vi "Reconstruct Installation Directory.vi"(10 "Build Type":string, 11 "Aliased Installation Path":path) -> (2 "NIPKG Directory":path, 3 "Real Installation Path":path)   [LabVIEW 2019, in "NIPKG Packager.lvclass"]
uses:
  NIPKG Packager.lvclass
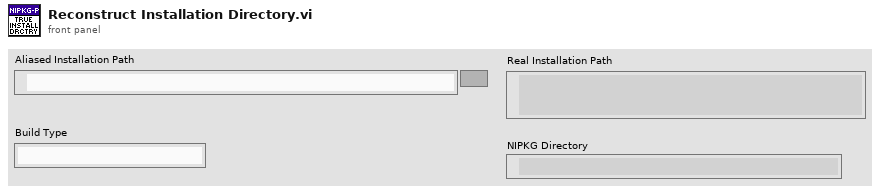
[diagram p1: front panel]
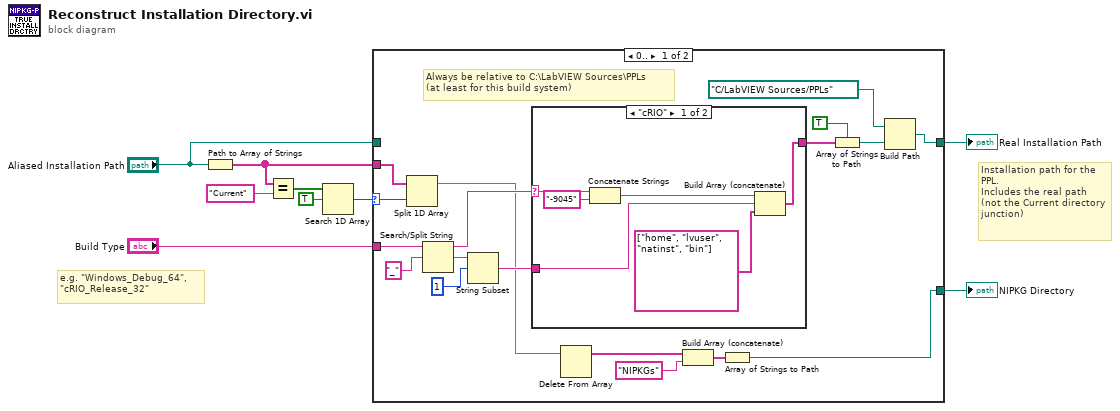
[diagram p0: block diagram]
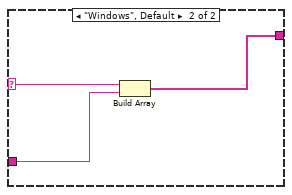
[diagram p2: hidden frame]
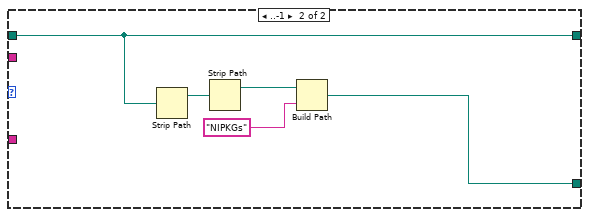
[diagram p3: hidden frame]
diagram:
  # "e.g. \"Windows_Debug_64\", \"cRIO_Release_32\""
  # "Installation path for the PPL.\nIncludes the real path (not the Current directory junction)"
  n1 = Path to Array of Strings(0:"Aliased Installation Path") -> (2:w3:string[])  [unwired: 1 out]
  n2 = Equal?(x=w3, y="Current") -> (x = y?=w8:bool[])
  n3 = Search 1D Array(1D array=w8, element=TRUE) -> (index of element=w6:i32)  [unwired: 1 in]
  n4 = case shown="0.." w6 {
    selector: w6 -> [w26 _]
    tunnel: [w11 w37] -> w5
    tunnel: "Build Type" -> [w24 _]
    tunnel: w3 -> [w27 _]
    tunnel: [w14 w38] -> w2
    tunnel: "Aliased Installation Path" -> [_ w37]
    frame 0.. {
      # "Always be relative to C:\\LabVIEW Sources\\PPLs\n(at least for this build system)"
      n5 = Split 1D Array(array=w27, index=w26) -> (first subarray=w18:string[])  [unwired: 1 out]
      n6 = Search/Split String(string=w24, search string/char (-)="_" ("delimiter")) -> (substring before match=w23:string, match + rest of string=w20:string)  [unwired: 1 in, 1 out]
      n7 = String Subset(string=w20, offset (0)=1) -> (substring=w19:string)  [unwired: 1 in]
      n8 = case shown="\"cRIO\"" w23 {
        selector: w23 -> [w32 w36]
        tunnel: [w28 w35] -> w22
        tunnel: w19 -> [w29 w34]
        frame "cRIO" {
          n9 = Concatenate Strings(w32, "-9045" ("string")) -> (w30:string)
          n10 = Build Array (concatenate)(w30, w29, string[] ["home", "lvuser", "natinst", "bin"] ("string")) -> (w28:string[])
        }
        frame "Windows", Default {
          n11 = Build Array(w36, w34) -> (w35:string[])
        }
      }
      n12 = Delete From Array(array=w18) -> (array with subset deleted=w17:string[])  [unwired: 2 in, 1 out]
      n13 = Build Array (concatenate)(w17, "NIPKGs") -> (w15:string[])
      n14 = Array of Strings to Path(0:w15) -> (2:w14:path)  [unwired: 1 in]
      n15 = Array of Strings to Path(0:w22, 1:TRUE ("relative")) -> (2:w12:path)
      n16 = Build Path(base path=path "C:/LabVIEW Sources/PPLs", name or relative path=w12) -> (appended path=w11:path)
    }
    frame ..-1 {
      n17 = Strip Path(path=w37) -> (stripped path=w41:path)  [unwired: 1 out]
      n18 = Strip Path(path=w41) -> (stripped path=w40:path)  [unwired: 1 out]
      n19 = Build Path(base path=w40, name or relative path="NIPKGs") -> (appended path=w38:path)
    }
  }
  "Real Installation Path" <- w5
  "NIPKG Directory" <- w2
